vi "Number to Proper English text - 0 to 99.vi"(8 "error in (no error)":errorcluster, 11 "Positive integer <= 99":u16) -> (0 "error out":errorcluster, 3 "Integer written in English":string)   [LabVIEW 2021, in "Project Euler.lvlib"]
uses:
  Project Euler.lvlib
panel:
  # "Development\ncontrols/indicators useful for development and testing, but which are not outputs of the VI"
  # "Input\nInputs to the VI"
  # "Output\nOutputs of the VI"
  # "Description\n\nBlank VI with error handling case. \n\nSummarize the use of this VI in this space."
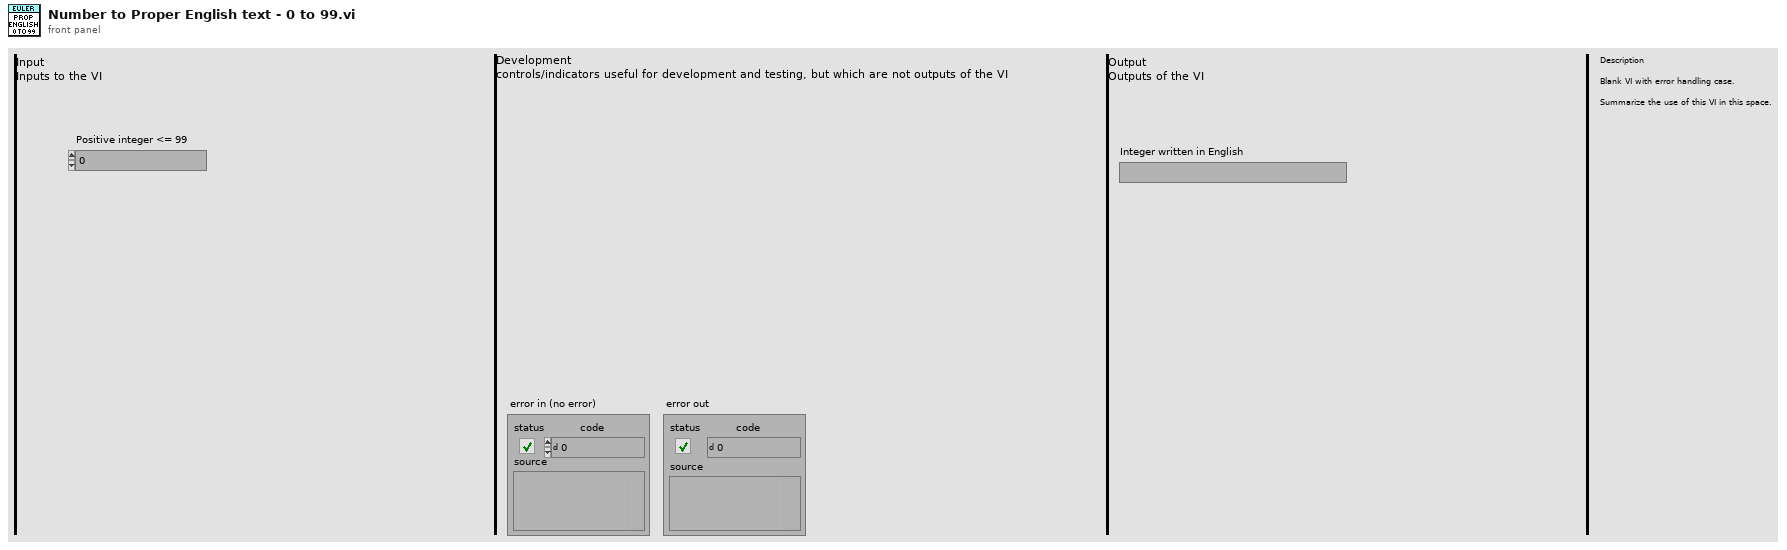
[diagram p1: front panel]
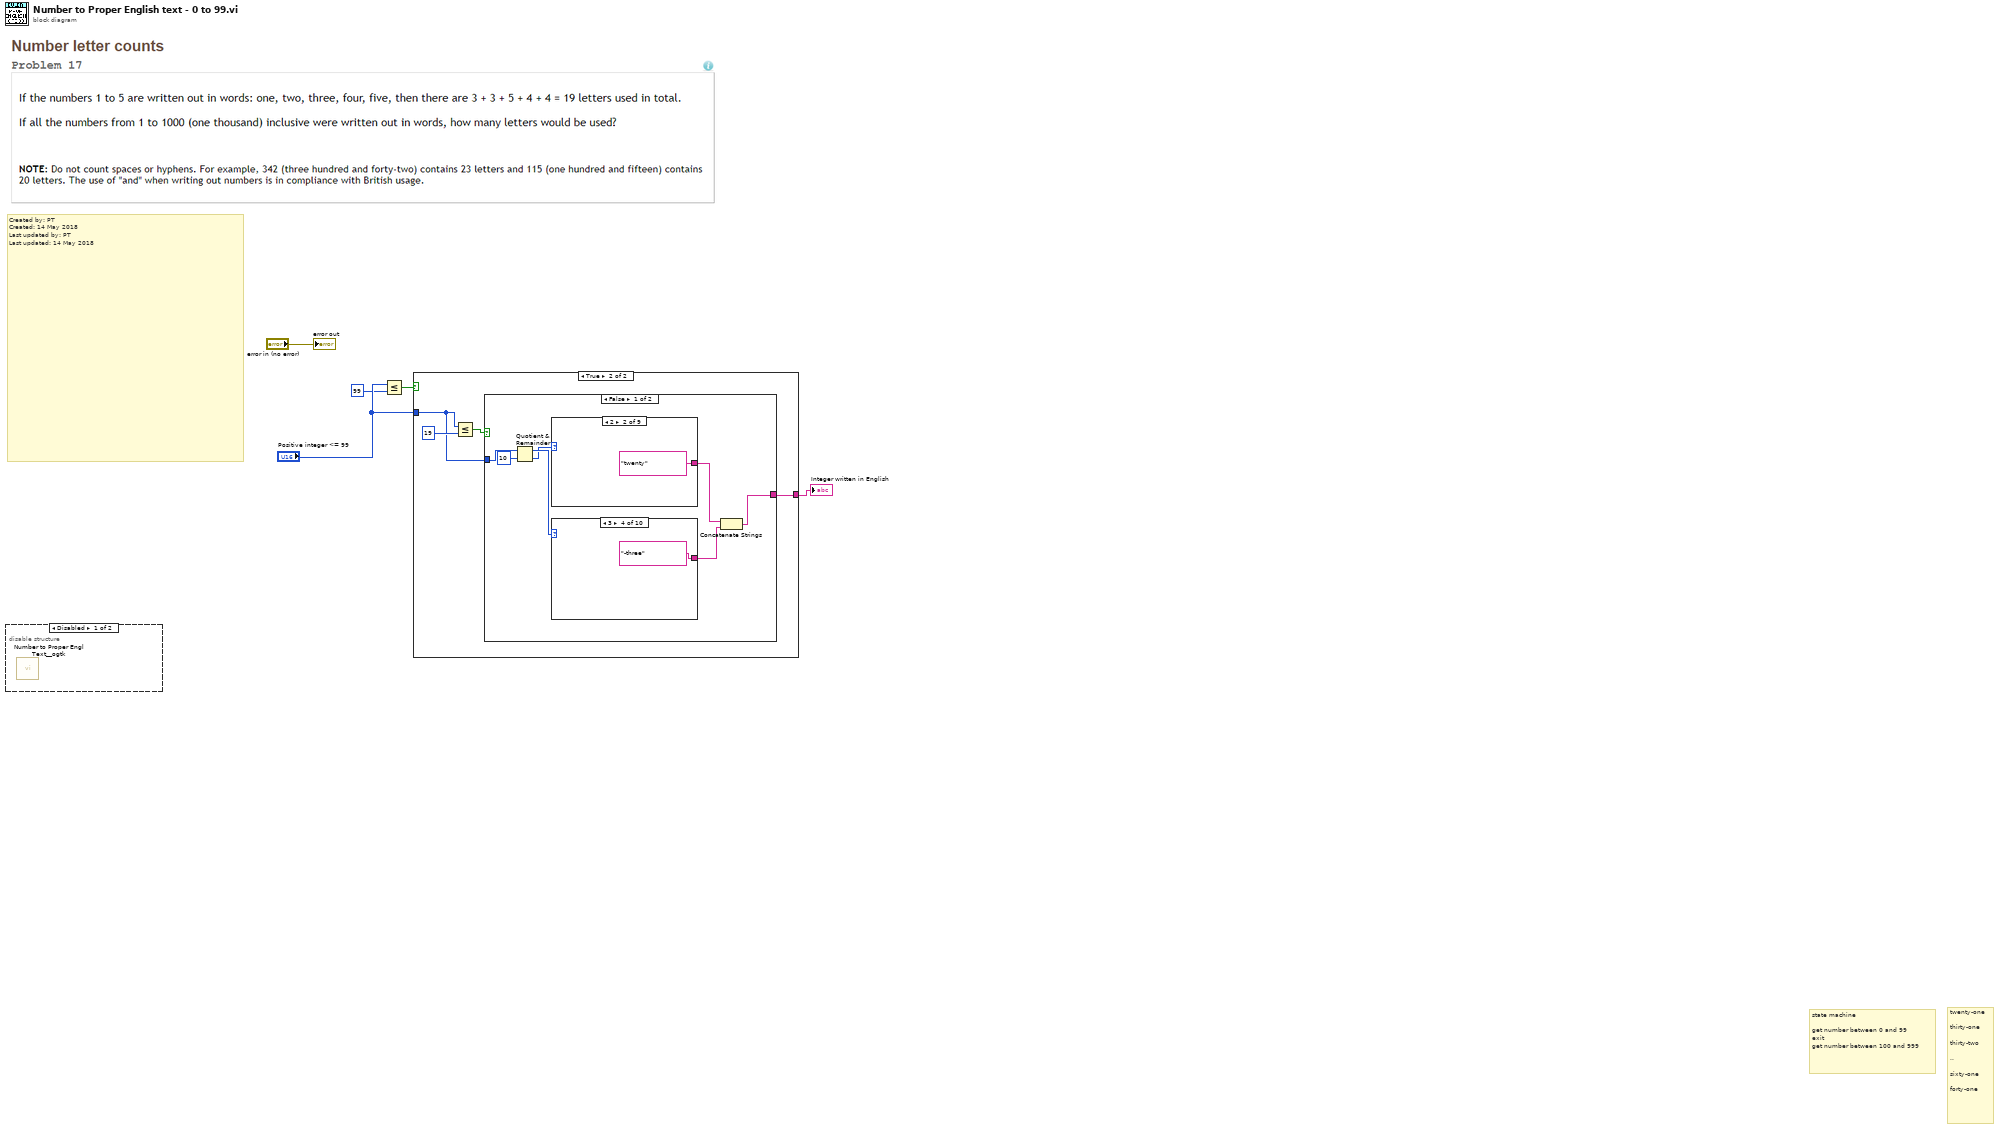
[diagram p0: block diagram]
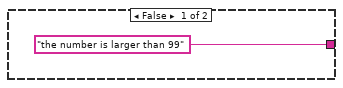
[diagram p2: hidden frame]
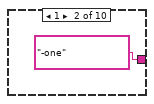
[diagram p4: hidden frame]
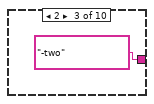
[diagram p5: hidden frame]
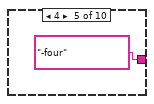
[diagram p6: hidden frame]
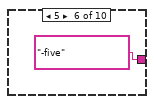
[diagram p7: hidden frame]
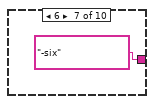
[diagram p8: hidden frame]
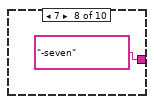
[diagram p9: hidden frame]
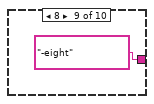
[diagram p10: hidden frame]
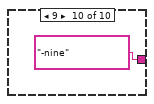
[diagram p11: hidden frame]
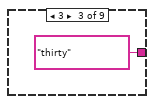
[diagram p13: hidden frame]
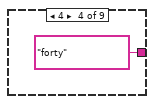
[diagram p14: hidden frame]
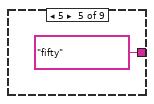
[diagram p15: hidden frame]
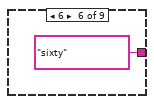
[diagram p16: hidden frame]
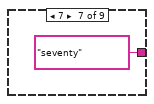
[diagram p17: hidden frame]
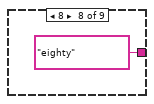
[diagram p18: hidden frame]
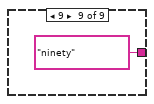
[diagram p19: hidden frame]
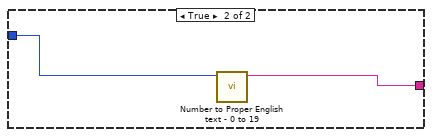
[diagram p20: hidden frame]
diagram:
  # "state machine\n\nget number between 0 and 99\nexit\nget number between 100 and 999"
  # "twenty-one\n\nthirty-one\n\nthirty-two\n\n..\n\nsixty-one\n\nforty-one"
  # "Created by: PT\nCreated: 14 May 2018\nLast updated by: PT\nLast updated: 14 May 2018"
  n1 = disable-structure shown="Disabled" {
    frame Disabled {
      n2 = call <userlib>:"Number to Proper Engl Text__ogtk.vi"() -> ()  [unwired: 5 in, 1 out]
    }
    frame Enabled {
    }
  }
  n3 = Less Or Equal?(x="Positive integer <= 99", y=u16 99) -> (x <= y?=w1:bool)
  n4 = case shown="True" w1 {
    tunnel: ["the number is larger than 99" w10] -> w4
    tunnel: "Positive integer <= 99" -> [_ w8]
    frame False {
    }
    frame True {
      n5 = Less Or Equal?(x=w8, y=u16 19) -> (x <= y?=w7:bool)
      n6 = case shown="False" w7 {
        tunnel: [w11 w35] -> w10
        tunnel: w8 -> [w12 w36]
        frame False {
          n7 = Quotient & Remainder(x=w12, y=u16 10) -> (x-y*floor(x/y)=w16:u16, floor(x/y)=w14:u16)
          n8 = case shown="2" w14 {
            tunnel: [_ "twenty" "thirty" "forty" "fifty" "sixty" "seventy" "eighty" "ninety"] -> w15
            frame Default {
            }
            frame 2 {
            }
            frame 3 {
            }
            frame 4 {
            }
            frame 5 {
            }
            frame 6 {
            }
            frame 7 {
            }
            frame 8 {
            }
            frame 9 {
            }
          }
          n9 = case shown="3" w16 {
            tunnel: [_ "-one" "-two" "-three" "-four" "-five" "-six" "-seven" "-eight" "-nine"] -> w17
            frame 0, Default {
            }
            frame 1 {
            }
            frame 2 {
            }
            frame 3 {
            }
            frame 4 {
            }
            frame 5 {
            }
            frame 6 {
            }
            frame 7 {
            }
            frame 8 {
            }
            frame 9 {
            }
          }
          n10 = Concatenate Strings(w15, w17) -> (w11:string)
        }
        frame True {
          n11 = call "Number to Proper English text - 0 to 19.vi"("Positive integer <= 19"=w36) -> ("Integer written in English"=w35:string)  [unwired: 9 in, 1 out]
        }
      }
    }
  }
  "Integer written in English" <- w4
  "error out" <- "error in (no error)"
